vi "GeoData.vi"() -> ()   [LabVIEW 2017] (continued)
31003\tClearwater\tNE\tAntelope County\tH1\n68764\t31003\tOrchard\tNE\tAntelope County\tH1\n68636\t31003\tElgin\tNE\tAntelope County\tH1\n68735\t31003\tEwing\tNE\tAntelope County\tH1\n68773\t31003\tRoyal\tNE\tAntelope County\tH1\n68761\t31003\tOakdale\tNE\tAntelope County\tH1\n68756\t31003\tNeligh\tNE\tAntelope County\tH1\n68729\t31003\tCreighton\tNE\tAntelope County\tH1\n69121\t31005\tArthur\tNE\tArthur County\tH1\n69146\t31005\tLemoyne\tNE\tArthur County\tH1\n69350\t31005\tHyannis\tNE\tArthur County\tH1\n69165\t31005\tSutherland\tNE\tArthur County\tH1\n69147\t31005\tLewellen\tNE\tArthur County\tH1\n69144\t31005\tKeystone\tNE\tArthur County\tH1\n69366\t31005\tWhitman\tNE\tArthur County\tH1\n69156\t31007\tPotter\tNE\tBanner County\tH1\n69145\t31007\tKimball\tNE\tBanner County\tH1\n69345\t31007\tHarrisburg\tNE\tBanner County\tH1\n69334\t31007\tBayard\tNE\tBanner County\tH1\n68833\t31009\tDunning\tNE\tBlaine County\tH1\n69157\t31009\tPurdum\tNE\tBlaine County\tH1\n68821\t31009\tBrewster\tNE\tBlaine County\tH1\n69163\t31009\tStapleton\tNE\tBlaine County\tH1\n69142\t31009\tHalsey\tNE\tBlaine County\tH1\n68781\t31011\tTilden\tNE\tBoone County\tH1\n68652\t31011\tPetersburg\tNE\tBoone County\tH1\n68655\t31011\tPrimrose\tNE\tBoone County\tH1\n68623\t31011\tBelgrade\tNE\tBoone County\tH1\n68660\t31011\tSaint edward\tNE\tBoone County\tH1\n68620\t31011\tAlbion\tNE\tBoone County\tH1\n68636\t31011\tElgin\tNE\tBoone County\tH1\n68638\t31011\tFullerton\tNE\tBoone County\tH1\n68627\t31011\tCedar rapids\tNE\tBoone County\tH1\n68758\t31011\tNewman grove\tNE\tBoone County\tH1\n68882\t31011\tWolbach\tNE\tBoone County\tH1\n69301\t31013\tAlliance\tNE\tBox Butte County\tH1\n69348\t31013\tHemingford\tNE\tBox Butte County\tH1\n69354\t31013\tMarsland\tNE\tBox Butte County\tH1\n68746\t31015\tLynch\tNE\tBoyd County\tH1\n68755\t31015\tNaper\tNE\tBoyd County\tH1\n68777\t31015\tSpencer\tNE\tBoyd County\tH1\n68722\t31015\tButte\tNE\tBoyd County\tH1\n68719\t31015\tBristow\tNE\tBoyd County\tH1\n68714\t31017\tBassett\tNE\tBrown County\tH1\n69210\t31017\tAinsworth\tNE\tBrown County\tH1\n69217\t31017\tLong pine\tNE\tBrown County\tH1\n69135\t31017\tElsmere\tNE\tBrown County\tH1\n69214\t31017\tJohnstown\tNE\tBrown County\tH1\n69221\t31017\tWood lake\tNE\tBrown County\tH1\n68847\t31019\tKearney\tNE\tBuffalo County\tH1\n68844\t31019\tHazard\tNE\tBuffalo County\tH1\n68956\t31019\tKenesaw\tNE\tBuffalo County\tH1\n68866\t31019\tPleasanton\tNE\tBuffalo County\tH1\n68947\t31019\tHildreth\tNE\tBuffalo County\tH1\n68845\t31019\tKearney\tNE\tBuffalo County\tH1\n68836\t31019\tElm creek\tNE\tBuffalo County\tH1\n68855\t31019\tMason city\tNE\tBuffalo County\tH1\n68876\t31019\tShelton\tNE\tBuffalo County\tH1\n68861\t31019\tOdessa\tNE\tBuffalo County\tH1\n68870\t31019\tRiverdale\tNE\tBuffalo County\tH1\n68840\t31019\tGibbon\tNE\tBuffalo County\tH1\n68849\t31019\tKearney\tNE\tBuffalo County\tH1\n68869\t31019\tRavenna\tNE\tBuffalo County\tH1\n68848\t31019\tKearney\tNE\tBuffalo County\tH1\n68858\t31019\tMiller\tNE\tBuffalo County\tH1\n68812\t31019\tAmherst\tNE\tBuffalo County\tH1\n68029\t31021\tHerman\tNE\tBurt County\tH1\n68019\t31021\tCraig\tNE\tBurt County\tH1\n68004\t31021\tBancroft\tNE\tBurt County\tH1\n68061\t31021\tTekamah\tNE\tBurt County\tH1\n68045\t31021\tOakland\tNE\tBurt County\tH1\n68031\t31021\tHooper\tNE\tBurt County\tH1\n68038\t31021\tLyons\tNE\tBurt County\tH1\n68020\t31021\tDecatur\tNE\tBurt County\tH1\n68036\t31023\tLinwood\tNE\tButler County\tH1\n68601\t31023\tColumbus\tNE\tButler County\tH1\n68626\t31023\tBrainard\tNE\tButler County\tH1\n68014\t31023\tBruno\tNE\tButler County\tH1\n68635\t31023\tDwight\tNE\tButler County\tH1\n68632\t31023\tDavid city\tNE\tButler County\tH1\n68658\t31023\tRising city\tNE\tButler County\tH1\n68669\t31023\tUlysses\tNE\tButler County\tH1\n68314\t31023\tBee\tNE\tButler County\tH1\n68662\t31023\tShelby\tNE\tButler County\tH1\n68001\t31023\tAbie\tNE\tButler County\tH1\n68624\t31023\tBellwood\tNE\tButler County\tH1\n68667\t31023\tSurprise\tNE\tButler County\tH1\n68349\t31025\tElmwood\tNE\tCass County\tH1\n68407\t31025\tMurdock\tNE\tCass County\tH1\n68016\t31025\tCedar creek\tNE\tCass County\tH1\n68037\t31025\tLouisville\tNE\tCass County\tH1\n68403\t31025\tManley\tNE\tCass County\tH1\n68347\t31025\tEagle\tNE\tCass County\tH1\n68454\t31025\tUnadilla\tNE\tCass County\tH1\n68058\t31025\tSouth bend\tNE\tCass County\tH1\n68048\t31025\tPlattsmouth\tNE\tCass County\tH1\n68527\t31025\tLincoln\tNE\tCass County\tH1\n68003\t31025\tAshland\tNE\tCass County\tH1\n68462\t31025\tWaverly\tNE\tCass County\tH1\n68304\t31025\tAlvo\tNE\tCass County\tH1\n68413\t31025\tNehawka\tNE\tCass County\tH1\n68455\t31025\tUnion\tNE\tCass County\tH1\n68418\t31025\tPalmyra\tNE\tCass County\tH1\n68307\t31025\tAvoca\tNE\tCass County\tH1\n68463\t31025\tWeeping water\tNE\tCass County\tH1\n68366\t31025\tGreenwood\tNE\tCass County\tH1\n68409\t31025\tMurray\tNE\tCass County\tH1\n68745\t31027\tLaurel\tNE\tCedar County\tH1\n68736\t31027\tFordyce\tNE\tCedar County\tH1\n68717\t31027\tBelden\tNE\tCedar County\tH1\n68786\t31027\tWausa\tNE\tCedar County\tH1\n68727\t31027\tColeridge\tNE\tCedar County\tH1\n68757\t31027\tNewcastle\tNE\tCedar County\tH1\n68739\t31027\tHartington\tNE\tCedar County\tH1\n68749\t31027\tMagnet\tNE\tCedar County\tH1\n68792\t31027\tWynot\tNE\tCedar County\tH1\n68771\t31027\tRandolph\tNE\tCedar County\tH1\n68774\t31027\tSaint helena\tNE\tCedar County\tH1\n68718\t31027\tBloomfield\tNE\tCedar County\tH1\n68730\t31027\tCrofton\tNE\tCedar County\tH1\n69027\t31029\tEnders\tNE\tChase County\tH1\n69030\t31029\tHaigler\tNE\tChase County\tH1\n69134\t31029\tElsie\tNE\tChase County\tH1\n69045\t31029\tWauneta\tNE\tChase County\tH1\n69033\t31029\tImperial\tNE\tChase County\tH1\n69023\t31029\tChampion\tNE\tChase County\tH1\n69168\t31029\tVenango\tNE\tChase County\tH1\n69343\t31031\tGordon\tNE\tCherry County\tH1\n69166\t31031\tThedford\tNE\tCherry County\tH1\n69212\t31031\tCrookston\tNE\tCherry County\tH1\n69211\t31031\tCody\tNE\tCherry County\tH1\n69350\t31031\tHyannis\tNE\tCherry County\tH1\n69219\t31031\tNenzel\tNE\tCherry County\tH1\n69220\t31031\tSparks\tNE\tCherry County\tH1\n69333\t31031\tAshby\tNE\tCherry County\tH1\n69161\t31031\tSeneca\tNE\tCherry County\tH1\n69201\t31031\tValentine\tNE\tCherry County\tH1\n69216\t31031\tKilgore\tNE\tCherry County\tH1\n69218\t31031\tMerriman\tNE\tCherry County\tH1\n69366\t31031\tWhitman\tNE\tCherry County\tH1\n69221\t31031\tWood lake\tNE\tCherry County\tH1\n69156\t31033\tPotter\tNE\tCheyenne County\tH1\n69149\t31033\tLodgepole\tNE\tCheyenne County\tH1\n69162\t31033\tSidney\tNE\tCheyenne County\tH1\n69141\t31033\tGurley\tNE\tCheyenne County\tH1\n69131\t31033\tDalton\tNE\tCheyenne County\tH1\n68436\t31035\tShickley\tNE\tClay County\tH1\n68452\t31035\tOng\tNE\tClay County\tH1\n68944\t31035\tHarvard\tNE\tClay County\tH1\n68933\t31035\tClay center\tNE\tClay County\tH1\n68935\t31035\tEdgar\tNE\tClay County\tH1\n68930\t31035\tBlue hill\tNE\tClay County\tH1\n68818\t31035\tAurora\tNE\tClay County\tH1\n68979\t31035\tSutton\tNE\tClay County\tH1\n68934\t31035\tDeweese\tNE\tClay County\tH1\n68901\t31035\tHastings\tNE\tClay County\tH1\n68941\t31035\tGlenvil\tNE\tClay County\tH1\n68975\t31035\tSaronville\tNE\tClay County\tH1\n68938\t31035\tFairfield\tNE\tClay County\tH1\n68954\t31035\tInland\tNE\tClay County\tH1\n68980\t31035\tTrumbull\tNE\tClay County\tH1\n68601\t31037\tColumbus\tNE\tColfax County\tH1\n68641\t31037\tHowells\tNE\tColfax County\tH1\n68659\t31037\tRogers\tNE\tColfax County\tH1\n68661\t31037\tSchuyler\tNE\tColfax County\tH1\n68643\t31037\tLeigh\tNE\tColfax County\tH1\n68633\t31037\tDodge\tNE\tColfax County\tH1\n68629\t31037\tClarkson\tNE\tColfax County\tH1\n68047\t31039\tPender\tNE\tCuming County\tH1\n68641\t31039\tHowells\tNE\tCuming County\tH1\n68004\t31039\tBancroft\tNE\tCuming County\tH1\n68045\t31039\tOakland\tNE\tCuming County\tH1\n68788\t31039\tWest point\tNE\tCuming County\tH1\n68716\t31039\tBeemer\tNE\tCuming County\tH1\n68768\t31039\tPilger\tNE\tCuming County\tH1\n68791\t31039\tWisner\tNE\tCuming County\tH1\n68633\t31039\tDodge\tNE\tCuming County\tH1\n68038\t31039\tLyons\tNE\tCuming County\tH1\n68825\t31041\tCallaway\tNE\tCuster County\tH1\n68856\t31041\tMerna\tNE\tCuster County\tH1\n69138\t31041\tGothenburg\tNE\tCuster County\tH1\n68833\t31041\tDunning\tNE\tCuster County\tH1\n68866\t31041\tPleasanton\tNE\tCuster County\tH1\n68815\t31041\tArcadia\tNE\tCuster County\tH1\n68860\t31041\tOconto\tNE\tCuster County\tH1\n68855\t31041\tMason city\tNE\tCuster County\tH1\n68881\t31041\tWesterville\tNE\tCuster County\tH1\n68874\t31041\tSargent\tNE\tCuster County\tH1\n68834\t31041\tEddyville\tNE\tCuster County\tH1\n68813\t31041\tAnselmo\tNE\tCuster County\tH1\n68850\t31041\tLexington\tNE\tCuster County\tH1\n68814\t31041\tAnsley\tNE\tCuster County\tH1\n68878\t31041\tSumner\tNE\tCuster County\tH1\n69120\t31041\tArnold\tNE\tCuster County\tH1\n68823\t31041\tBurwell\tNE\tCuster County\tH1\n68852\t31041\tLitchfield\tNE\tCuster County\tH1\n68822\t31041\tBroken bow\tNE\tCuster County\tH1\n68828\t31041\tComstock\tNE\tCuster County\tH1\n68030\t31043\tHomer\tNE\tDakota County\tH1\n68741\t31043\tHubbard\tNE\tDakota County\tH1\n68731\t31043\tDakota city\tNE\tDakota County\tH1\n68770\t31043\tPonca\tNE\tDakota County\tH1\n68733\t31043\tEmerson\tNE\tDakota County\tH1\n68776\t31043\tSouth sioux city\tNE\tDakota County\tH1\n68743\t31043\tJackson\tNE\tDakota County\tH1\n68785\t31043\tWaterbury\tNE\tDakota County\tH1\n69348\t31045\tHemingford\tNE\tDawes County\tH1\n69337\t31045\tChadron\tNE\tDawes County\tH1\n69347\t31045\tHay springs\tNE\tDawes County\tH1\n69339\t31045\tCrawford\tNE\tDawes County\tH1\n69367\t31045\tWhitney\tNE\tDawes County\tH1\n69354\t31045\tMarsland\tNE\tDawes County\tH1\n69029\t31047\tFarnam\tNE\tDawson County\tH1\n69138\t31047\tGothenburg\tNE\tDawson County\tH1\n68836\t31047\tElm creek\tNE\tDawson County\tH1\n69130\t31047\tCozad\tNE\tDawson County\tH1\n69171\t31047\tWillow island\tNE\tDawson County\tH1\n68834\t31047\tEddyville\tNE\tDawson County\tH1\n69028\t31047\tEustis\tNE\tDawson County\tH1\n68850\t31047\tLexington\tNE\tDawson County\tH1\n68878\t31047\tSumner\tNE\tDawson County\tH1\n68863\t31047\tOverton\tNE\tDawson County\tH1\n68937\t31047\tElwood\tNE\tDawson County\tH1\n68858\t31047\tMiller\tNE\tDawson County\tH1\n69129\t31049\tChappell\tNE\tDeuel County\tH1\n69149\t31049\tLodgepole\tNE\tDeuel County\tH1\n69122\t31049\tBig springs\tNE\tDeuel County\tH1\n68745\t31051\tLaurel\tNE\tDixon County\tH1\n68757\t31051\tNewcastle\tNE\tDixon County\tH1\n68739\t31051\tHartington\tNE\tDixon County\tH1\n68770\t31051\tPonca\tNE\tDixon County\tH1\n68733\t31051\tEmerson\tNE\tDixon County\tH1\n68732\t31051\tDixon\tNE\tDixon County\tH1\n68792\t31051\tWynot\tNE\tDixon County\tH1\n68787\t31051\tWayne\tNE\tDixon County\tH1\n68710\t31051\tAllen\tNE\tDixon County\tH1\n68728\t31051\tConcord\tNE\tDixon County\tH1\n68784\t31051\tWakefield\tNE\tDixon County\tH1\n68785\t31051\tWaterbury\tNE\tDixon County\tH1\n68751\t31051\tMaskell\tNE\tDixon County\tH1\n68063\t31053\tUehling\tNE\tDodge County\tH1\n68026\t31053\tFremont\tNE\tDodge County\tH1\n68044\t31053\tNickerson\tNE\tDodge County\tH1\n68064\t31053\tValley\tNE\tDodge County\tH1\n68045\t31053\tOakland\tNE\tDodge County\tH1\n68649\t31053\tNorth bend\tNE\tDodge County\tH1\n68788\t31053\tWest point\tNE\tDodge County\tH1\n68664\t31053\tSnyder\tNE\tDodge County\tH1\n68025\t31053\tFremont\tNE\tDodge County\tH1\n68621\t31053\tAmes\tNE\tDodge County\tH1\n68031\t31053\tHooper\tNE\tDodge County\tH1\n68072\t31053\tWinslow\tNE\tDodge County\tH1\n68633\t31053\tDodge\tNE\tDodge County\tH1\n68057\t31053\tScribner\tNE\tDodge County\tH1\n68118\t31055\tOmaha\tNE\tDouglas County\tH1\n68106\t31055\tOmaha\tNE\tDouglas County\tH1\n68022\t31055\tElkhorn\tNE\tDouglas County\tH1\n68135\t31055\tOmaha\tNE\tDouglas County\tH1\n68117\t31055\tOmaha\tNE\tDouglas County\tH1\n68108\t31055\tOmaha\tNE\tDouglas County\tH1\n68137\t31055\tOmaha\tNE\tDouglas County\tH1\n68154\t31055\tOmaha\tNE\tDouglas County\tH1\n68152\t31055\tOmaha\tNE\tDouglas County\tH1\n68007\t31055\tBennington\tNE\tDouglas County\tH1\n68182\t31055\tOmaha\tNE\tDouglas County\tH1\n68112\t31055\tOmaha\tNE\tDouglas County\tH1\n68114\t31055\tOmaha\tNE\tDouglas County\tH1\n68116\t31055\tOmaha\tNE\tDouglas County\tH1\n68127\t31055\tOmaha\tNE\tDouglas County\tH1\n68138\t31055\tOmaha\tNE\tDouglas County\tH1\n68197\t31055\tOmaha\tNE\tDouglas County\tH1\n68145\t31055\tOmaha\tNE\tDouglas County\tH1\n68179\t31055\tOmaha\tNE\tDouglas County\tH1\n68139\t31055\tOmaha\tNE\tDouglas County\tH1\n68175\t31055\tOmaha\tNE\tDouglas County\tH1\n68122\t31055\tOmaha\tNE\tDouglas County\tH1\n68102\t31055\tOmaha\tNE\tDouglas County\tH1\n68064\t31055\tValley\tNE\tDouglas County\tH1\n68136\t31055\tOmaha\tNE\tDouglas County\tH1\n68069\t31055\tWaterloo\tNE\tDouglas County\tH1\n68198\t31055\tOmaha\tNE\tDouglas County\tH1\n68111\t31055\tOmaha\tNE\tDouglas County\tH1\n68144\t31055\tOmaha\tNE\tDouglas County\tH1\n68130\t31055\tOmaha\tNE\tDouglas County\tH1\n68109\t31055\tOmaha\tNE\tDouglas County\tH1\n68134\t31055\tOmaha\tNE\tDouglas County\tH1\n68107\t31055\tOmaha\tNE\tDouglas County\tH1\n68110\t31055\tOmaha\tNE\tDouglas County\tH1\n68131\t31055\tOmaha\tNE\tDouglas County\tH1\n68147\t31055\tBellevue\tNE\tDouglas County\tH1\n68010\t31055\tBoys town\tNE\tDouglas County\tH1\n68180\t31055\tOmaha\tNE\tDouglas County\tH1\n68178\t31055\tOmaha\tNE\tDouglas County\tH1\n68105\t31055\tOmaha\tNE\tDouglas County\tH1\n68124\t31055\tOmaha\tNE\tDouglas County\tH1\n68132\t31055\tOmaha\tNE\tDouglas County\tH1\n68142\t31055\tOmaha\tNE\tDouglas County\tH1\n68103\t31055\tOmaha\tNE\tDouglas County\tH1\n68028\t31055\tGretna\tNE\tDouglas County\tH1\n68104\t31055\tOmaha\tNE\tDouglas County\tH1\n68128\t31055\tLa vista\tNE\tDouglas County\tH1\n68164\t31055\tOmaha\tNE\tDouglas County\tH1\n68157\t31055\tOmaha\tNE\tDouglas County\tH1\n68183\t31055\tOmaha\tNE\tDouglas County\tH1\n69037\t31057\tMax\tNE\tDundy County\tH1\n69027\t31057\tEnders\tNE\tDundy County\tH1\n69030\t31057\tHaigler\tNE\tDundy County\tH1\n69045\t31057\tWauneta\tNE\tDundy County\tH1\n69021\t31057\tBenkelman\tNE\tDundy County\tH1\n69041\t31057\tParks\tNE\tDundy County\tH1\n68436\t31059\tShickley\tNE\tFillmore County\tH1\n68452\t31059\tOng\tNE\tFillmore County\tH1\n68444\t31059\tStrang\tNE\tFillmore County\tH1\n68416\t31059\tOhiowa\tNE\tFillmore County\tH1\n68326\t31059\tCarleton\tNE\tFillmore County\tH1\n68406\t31059\tMilligan\tNE\tFillmore County\tH1\n68361\t31059\tGeneva\tNE\tFillmore County\tH1\n68359\t31059\tFriend\tNE\tFillmore County\tH1\n68351\t31059\tExeter\tNE\tFillmore County\tH1\n68354\t31059\tFairmont\tNE\tFillmore County\tH1\n68979\t31059\tSutton\tNE\tFillmore County\tH1\n68365\t31059\tGrafton\tNE\tFillmore County\tH1\n68322\t31059\tBruning\tNE\tFillmore County\tH1\n68335\t31059\tDavenport\tNE\tFillmore County\tH1\n68972\t31061\tRiverton\tNE\tFranklin County\tH1\n68947\t31061\tHildreth\tNE\tFranklin County\tH1\n68939\t31061\tFranklin\tNE\tFranklin County\tH1\n68981\t31061\tUpland\tNE\tFranklin County\tH1\n68982\t31061\tWilcox\tNE\tFranklin County\tH1\n68960\t31061\tNaponee\tNE\tFranklin County\tH1\n68932\t31061\tCampbell\tNE\tFranklin County\tH1\n68952\t31061\tInavale\tNE\tFranklin County\tH1\n68929\t31061\tBloomington\tNE\tFranklin County\tH1\n69029\t31063\tFarnam\tNE\tFrontier County\tH1\n69038\t31063\tMaywood\tNE\tFrontier County\tH1\n69039\t31063\tMoorefield\tNE\tFrontier County\tH1\n69001\t31063\tMc cook\tNE\tFrontier County\tH1\n69022\t31063\tCambridge\tNE\tFrontier County\tH1\n69028\t31063\tEustis\tNE\tFrontier County\tH1\n68948\t31063\tHolbrook\tNE\tFrontier County\tH1\n69025\t31063\tCurtis\tNE\tFrontier County\tH1\n69042\t31063\tStockville\tNE\tFrontier County\tH1\n69034\t31063\tIndianola\tNE\tFrontier County\tH1\n68922\t31065\tArapahoe\tNE\tFurnas County\tH1\n68977\t31065\tStamford\tNE\tFurnas County\tH1\n68936\t31065\tEdison\tNE\tFurnas County\tH1\n69022\t31065\tCambridge\tNE\tFurnas County\tH1\n69046\t31065\tWilsonville\tNE\tFurnas County\tH1\n68967\t31065\tOxford\tNE\tFurnas County\tH1\n69020\t31065\tBartley\tNE\tFurnas County\tH1\n68926\t31065\tBeaver city\tNE\tFurnas County\tH1\n68948\t31065\tHolbrook\tNE\tFurnas County\tH1\n68946\t31065\tHendley\tNE\tFurnas County\tH1\n68309\t31067\tBarneston\tNE\tGage County\tH1\n68301\t31067\tAdams\tNE\tGage County\tH1\n68458\t31067\tVirginia\tNE\tGage County\tH1\n68331\t31067\tCortland\tNE\tGage County\tH1\n68342\t31067\tDiller\tNE\tGage County\tH1\n68422\t31067\tPickrell\tNE\tGage County\tH1\n68323\t31067\tBurchard\tNE\tGage County\tH1\n68466\t31067\tWymore\tNE\tGage County\tH1\n68368\t31067\tHallam\tNE\tGage County\tH1\n68381\t31067\tLiberty\tNE\tGage County\tH1\n68328\t31067\tClatonia\tNE\tGage County\tH1\n68341\t31067\tDe witt\tNE\tGage County\tH1\n68404\t31067\tMartell\tNE\tGage County\tH1\n68332\t31067\tCrab orchard\tNE\tGage County\tH1\n68415\t31067\tOdell\tNE\tGage County\tH1\n68465\t31067\tWilber\tNE\tGage County\tH1\n68358\t31067\tFirth\tNE\tGage County\tH1\n68310\t31067\tBeatrice\tNE\tGage County\tH1\n68318\t31067\tBlue springs\tNE\tGage County\tH1\n68424\t31067\tPlymouth\tNE\tGage County\tH1\n68357\t31067\tFilley\tNE\tGage County\tH1\n69129\t31069\tChappell\tNE\tGarden County\tH1\n69351\t31069\tLakeside\tNE\tGarden County\tH1\n69335\t31069\tBingham\tNE\tGarden County\tH1\n69149\t31069\tLodgepole\tNE\tGarden County\tH1\n69333\t31069\tAshby\tNE\tGarden County\tH1\n69148\t31069\tLisco\tNE\tGarden County\tH1\n69190\t31069\tOshkosh\tNE\tGarden County\tH1\n69147\t31069\tLewellen\tNE\tGarden County\tH1\n69154\t31069\tOshkosh\tNE\tGarden County\tH1\n69122\t31069\tBig springs\tNE\tGarden County\tH1\n69340\t31069\tEllsworth\tNE\tGarden County\tH1\n68725\t31071\tChambers\tNE\tGarfield County\tH1\n68862\t31071\tOrd\tNE\tGarfield County\tH1\n68823\t31071\tBurwell\tNE\tGarfield County\tH1\n68637\t31071\tEricson\tNE\tGarfield County\tH1\n68922\t31073\tArapahoe\tNE\tGosper County\tH1\n68936\t31073\tEdison\tNE\tGosper County\tH1\n69022\t31073\tCambridge\tNE\tGosper County\tH1\n68967\t31073\tOxford\tNE\tGosper County\tH1\n69028\t31073\tEustis\tNE\tGosper County\tH1\n68850\t31073\tLexington\tNE\tGosper County\tH1\n68937\t31073\tElwood\tNE\tGosper County\tH1\n68948\t31073\tHolbrook\tNE\tGosper County\tH1\n68927\t31073\tBertrand\tNE\tGosper County\tH1\n68976\t31073\tSmithfield\tNE\tGosper County\tH1\n69350\t31075\tHyannis\tNE\tGrant County\tH1\n69333\t31075\tAshby\tNE\tGrant County\tH1\n69366\t31075\tWhitman\tNE\tGrant County\tH1\n68835\t31077\tElba\tNE\tGreeley County\tH1\n68665\t31077\tSpalding\tNE\tGreeley County\tH1\n68655\t31077\tPrimrose\tNE\tGreeley County\tH1\n68842\t31077\tGreeley\tNE\tGreeley County\tH1\n68875\t31077\tScotia\tNE\tGreeley County\tH1\n68637\t31077\tEricson\tNE\tGreeley County\tH1\n68859\t31077\tNorth loup\tNE\tGreeley County\tH1\n68627\t31077\tCedar rapids\tNE\tGreeley County\tH1\n68882\t31077\tWolbach\tNE\tGreeley County\tH1\n68955\t31079\tJuniata\tNE\tHall County\tH1\n68956\t31079\tKenesaw\tNE\tHall County\tH1\n68831\t31079\tDannebrog\tNE\tHall County\tH1\n68876\t31079\tShelton\tNE\tHall County\tH1\n68865\t31079\tPhillips\tNE\tHall County\tH1\n68832\t31079\tDoniphan\tNE\tHall County\tH1\n68810\t31079\tAlda\tNE\tHall County\tH1\n68883\t31079\tWood river\tNE\tHall County\tH1\n68803\t31079\tGrand island\tNE\tHall County\tH1\n68802\t31079\tGrand island\tNE\tHall County\tH1\n68901\t31079\tHastings\tNE\tHall County\tH1\n68824\t31079\tCairo\tNE\tHall County\tH1\n68869\t31079\tRavenna\tNE\tHall County\tH1\n68872\t31079\tSaint libory\tNE\tHall County\tH1\n68801\t31079\tGrand island\tNE\tHall County\tH1\n68980\t31079\tTrumbull\tNE\tHall County\tH1\n68654\t31081\tPolk\tNE\tHamilton County\tH1\n68944\t31081\tHarvard\tNE\tHamilton County\tH1\n68854\t31081\tMarquette\tNE\tHamilton County\tH1\n68628\t31081\tClarks\tNE\tHamilton County\tH1\n68371\t31081\tHenderson\tNE\tHamilton County\tH1\n68865\t31081\tPhillips\tNE\tHamilton County\tH1\n68832\t31081\tDoniphan\tNE\tHamilton County\tH1\n68846\t31081\tHordville\tNE\tHamilton County\tH1\n68841\t31081\tGiltner\tNE\tHamilton County\tH1\n68319\t31081\tBradshaw\tNE\tHamilton County\tH1\n68818\t31081\tAurora\tNE\tHamilton County\tH1\n68979\t31081\tSutton\tNE\tHamilton County\tH1\n68843\t31081\tHampton\tNE\tHamilton County\tH1\n68980\t31081\tTrumbull\tNE\tHamilton County\tH1\n68977\t31083\tStamford\tNE\tHarlan County\tH1\n68949\t31083\tHoldrege\tNE\tHarlan County\tH1\n68967\t31083\tOxford\tNE\tHarlan County\tH1\n68920\t31083\tAlma\tNE\tHarlan County\tH1\n68982\t31083\tWilcox\tNE\tHarlan County\tH1\n68960\t31083\tNaponee\tNE\tHarlan County\tH1\n68966\t31083\tOrleans\tNE\tHarlan County\tH1\n68971\t31083\tRepublican city\tNE\tHarlan County\tH1\n68969\t31083\tRagan\tNE\tHarlan County\tH1\n69038\t31085\tMaywood\tNE\tHayes County\tH1\n69024\t31085\tCulbertson\tNE\tHayes County\tH1\n69169\t31085\tWallace\tNE\tHayes County\tH1\n69032\t31085\tHayes center\tNE\tHayes County\tH1\n69134\t31085\tElsie\tNE\tHayes County\tH1\n69045\t31085\tWauneta\tNE\tHayes County\tH1\n69040\t31085\tPalisade\tNE\tHayes County\tH1\n69038\t31087\tMaywood\tNE\tHitchcock County\tH1\n69024\t31087\tCulbertson\tNE\tHitchcock County\tH1\n69043\t31087\tStratton\tNE\tHitchcock County\tH1\n69001\t31087\tMc cook\tNE\tHitchcock County\tH1\n69045\t31087\tWauneta\tNE\tHitchcock County\tH1\n69040\t31087\tPalisade\tNE\tHitchcock County\tH1\n69044\t31087\tTrenton\tNE\tHitchcock County\tH1\n68766\t31089\tPage\tNE\tHolt County\tH1\n68759\t31089\tNewport\tNE\tHolt County\tH1\n68725\t31089\tChambers\tNE\tHolt County\tH1\n68713\t31089\tAtkinson\tNE\tHolt County\tH1\n68746\t31089\tLynch\tNE\tHolt County\tH1\n68726\t31089\tClearwater\tNE\tHolt County\tH1\n68823\t31089\tBurwell\tNE\tHolt County\tH1\n68764\t31089\tOrchard\tNE\tHolt County\tH1\n68735\t31089\tEwing\tNE\tHolt County\tH1\n68763\t31089\tOneill\tNE\tHolt County\tH1\n68711\t31089\tAmelia\tNE\tHolt County\tH1\n68777\t31089\tSpencer\tNE\tHolt County\tH1\n68780\t31089\tStuart\tNE\tHolt County\tH1\n68734\t31089\tEmmet\tNE\tHolt County\tH1\n68742\t31089\tInman\tNE\tHolt County\tH1\n69152\t31091\tMullen\tNE\tHooker County\tH1\n69167\t31091\tTryon\tNE\tHooker County\tH1\n68873\t31093\tSaint paul\tNE\tHoward County\tH1\n68816\t31093\tArcher\tNE\tHoward County\tH1\n68835\t31093\tElba\tNE\tHoward County\tH1\n68831\t31093\tDannebrog\tNE\tHoward County\tH1\n68817\t31093\tAshton\tNE\tHoward County\tH1\n68864\t31093\tPalmer\tNE\tHoward County\tH1\n68875\t31093\tScotia\tNE\tHoward County\tH1\n68838\t31093\tFarwell\tNE\tHoward County\tH1\n68803\t31093\tGrand island\tNE\tHoward County\tH1\n68824\t31093\tCairo\tNE\tHoward County\tH1\n68872\t31093\tSaint libory\tNE\tHoward County\tH1\n68801\t31093\tGrand island\tNE\tHoward County\tH1\n68882\t31093\tWolbach\tNE\tHoward County\tH1\n68820\t31093\tBoelus\tNE\tHoward County\tH1\n68352\t31095\tFairbury\tNE\tJefferson County\tH1\n68464\t31095\tWestern\tNE\tJefferson County\tH1\n68350\t31095\tEndicott\tNE\tJefferson County\tH1\n68342\t31095\tDiller\tNE\tJefferson County\tH1\n68440\t31095\tSteele city\tNE\tJefferson County\tH1\n68303\t31095\tAlexandria\tNE\tJefferson County\tH1\n68429\t31095\tReynolds\tNE\tJefferson County\tH1\n68341\t31095\tDe witt\tNE\tJefferson County\tH1\n68370\t31095\tHebron\tNE\tJefferson County\tH1\n68453\t31095\tTobias\tNE\tJefferson County\tH1\n68310\t31095\tBeatrice\tNE\tJefferson County\tH1\n68424\t31095\tPlymouth\tNE\tJefferson County\tH1\n68338\t31095\tDaykin\tNE\tJefferson County\tH1\n68377\t31095\tJansen\tNE\tJefferson County\tH1\n68301\t31097\tAdams\tNE\tJohnson County\tH1\n68378\t31097\tJohnson\tNE\tJohnson County\tH1\n68329\t31097\tCook\tNE\tJohnson County\tH1\n68443\t31097\tSterling\tNE\tJohnson County\tH1\n68450\t31097\tTecumseh\tNE\tJohnson County\tH1\n68324\t31097\tBurr\tNE\tJohnson County\tH1\n68332\t31097\tCrab orchard\tNE\tJohnson County\tH1\n68447\t31097\tTable rock\tNE\tJohnson County\tH1\n68348\t31097\tElk creek\tNE\tJohnson County\tH1\n68448\t31097\tTalmage\tNE\tJohnson County\tH1\n68847\t31099\tKearney\tNE\tKearney County\tH1\n68956\t31099\tKenesaw\tNE\tKearney County\tH1\n68972\t31099\tRiverton\tNE\tKearney County\tH1\n68945\t31099\tHeartwell\tNE\tKearney County\tH1\n68947\t31099\tHildreth\tNE\tKearney County\tH1\n68845\t31099\tKearney\tNE\tKearney County\tH1\n68924\t31099\tAxtell\tNE\tKearney County\tH1\n68939\t31099\tFranklin\tNE\tKearney County\tH1\n68981\t31099\tUpland\tNE\tKearney County\tH1\n68840\t31099\tGibbon\tNE\tKearney County\tH1\n68982\t31099\tWilcox\tNE\tKearney County\tH1\n68959\t31099\tMinden\tNE\tKearney County\tH1\n68932\t31099\tCampbell\tNE\tKearney County\tH1\n69121\t31101\tArthur\tNE\tKeith County\tH1\n69155\t31101\tPaxton\tNE\tKeith County\tH1\n69146\t31101\tLemoyne\tNE\tKeith County\tH1\n69153\t31101\tOgallala\tNE\tKeith County\tH1\n69165\t31101\tSutherland\tNE\tKeith County\tH1\n69147\t31101\tLewellen\tNE\tKeith County\tH1\n69144\t31101\tKeystone\tNE\tKeith County\tH1\n69127\t31101\tBrule\tNE\tKeith County\tH1\n69122\t31101\tBig springs\tNE\tKeith County\tH1\n68753\t31103\tMills\tNE\tKeya Paha County\tH1\n68778\t31103\tSpringview\tNE\tKeya Paha County\tH1\n69156\t31105\tPotter\tNE\tKimball County\tH1\n69145\t31105\tKimball\tNE\tKimball County\tH1\n69133\t31105\tDix\tNE\tKimball County\tH1\n69128\t31105\tBushnell\tNE\tKimball County\tH1\n68760\t31107\tNiobrara\tNE\tKnox County\tH1\n68769\t31107\tPlainview\tNE\tKnox County\tH1\n68786\t31107\tWausa\tNE\tKnox County\tH1\n68724\t31107\tCenter\tNE\tKnox County\tH1\n68789\t31107\tWinnetoon\tNE\tKnox County\tH1\n68783\t31107\tVerdigre\tNE\tKnox County\tH1\n68764\t31107\tOrchard\tNE\tKnox County\tH1\n68773\t31107\tRoyal\tNE\tKnox County\tH1\n68763\t31107\tOneill\tNE\tKnox County\tH1\n68718\t31107\tBloomfield\tNE\tKnox County\tH1\n68730\t31107\tCrofton\tNE\tKnox County\tH1\n68729\t31107\tCreighton\tNE\tKnox County\tH1\n68503\t31109\tLincoln\tNE\tLancaster County\tH1\n68428\t31109\tRaymond\tNE\tLancaster County\tH1\n68526\t31109\tLincoln\tNE\tLancaster County\tH1\n68301\t31109\tAdams\tNE\tLancaster County\tH1\n68419\t31109\tPanama\tNE\tLancaster County\tH1\n68017\t31109\tCeresco\tNE\tLancaster County\tH1\n68331\t31109\tCortland\tNE\tLancaster County\tH1\n68522\t31109\tLincoln\tNE\tLancaster County\tH1\n68523\t31109\tLincoln\tNE\tLancaster County\tH1\n68438\t31109\tSprague\tNE\tLancaster County\tH1\n68501\t31109\tLincoln\tNE\tLancaster County\tH1\n68339\t31109\tDenton\tNE\tLancaster County\tH1\n68360\t31109\tGarland\tNE\tLancaster County\tH1\n68065\t31109\tValparaiso\tNE\tLancaster County\tH1\n68502\t31109\tLincoln\tNE\tLancaster County\tH1\n68507\t31109\tLincoln\tNE\tLancaster County\tH1\n68423\t31109\tPleasant dale\tNE\tLancaster County\tH1\n68516\t31109\tLincoln\tNE\tLancaster County\tH1\n68528\t31109\tLincoln\tNE\tLancaster County\tH1\n68588\t31109\tLincoln\tNE\tLancaster County\tH1\n68347\t31109\tEagle\tNE\tLancaster County\tH1\n68368\t31109\tHallam\tNE\tLancaster County\tH1\n68506\t31109\tLincoln\tNE\tLancaster County\tH1\n68510\t31109\tLincoln\tNE\tLancaster County\tH1\n68527\t31109\tLincoln\tNE\tLancaster County\tH1\n68003\t31109\tAshland\tNE\tLancaster County\tH1\n68404\t31109\tMartell\tNE\tLancaster County\tH1\n68517\t31109\tLincoln\tNE\tLancaster County\tH1\n68529\t31109\tLincoln\tNE\tLancaster County\tH1\n68372\t31109\tHickman\tNE\tLancaster County\tH1\n68462\t31109\tWaverly\tNE\tLancaster County\tH1\n68333\t31109\tCrete\tNE\tLancaster County\tH1\n68402\t31109\tMalcolm\tNE\tLancaster County\tH1\n68524\t31109\tLincoln\tNE\tLancaster County\tH1\n68512\t31109\tLincoln\tNE\tLancaster County\tH1\n68465\t31109\tWilber\tNE\tLancaster County\tH1\n68317\t31109\tBennet\tNE\tLancaster County\tH1\n68358\t31109\tFirth\tNE\tLancaster County\tH1\n68514\t31109\tLincoln\tNE\tLancaster County\tH1\n68504\t31109\tLincoln\tNE\tLancaster County\tH1\n68505\t31109\tLincoln\tNE\tLancaster County\tH1\n68366\t31109\tGreenwood\tNE\tLancaster County\tH1\n68521\t31109\tLincoln\tNE\tLancaster County\tH1\n68532\t31109\tLincoln\tNE\tLancaster County\tH1\n68508\t31109\tLincoln\tNE\tLancaster County\tH1\n68520\t31109\tLincoln\tNE\tLancaster County\tH1\n68430\t31109\tRoca\tNE\tLancaster County\tH1\n68461\t31109\tWalton\tNE\tLancaster County\tH1\n68531\t31109\tLincoln\tNE\tLancaster County\tH1\n68336\t31109\tDavey\tNE\tLancaster County\tH1\n68542\t31109\tLincoln\tNE\tLancaster County\tH1\n69029\t31111\tFarnam\tNE\tLincoln County\tH1\n69101\t31111\tNorth platte\tNE\tLincoln County\tH1\n69138\t31111\tGothenburg\tNE\tLincoln County\tH1\n69038\t31111\tMaywood\tNE\tLincoln County\tH1\n69039\t31111\tMoorefield\tNE\tLincoln County\tH1\n69169\t31111\tWallace\tNE\tLincoln County\tH1\n69123\t31111\tBrady\tNE\tLincoln County\tH1\n69170\t31111\tWellfleet\tNE\tLincoln County\tH1\n69165\t31111\tSutherland\tNE\tLincoln County\tH1\n69103\t31111\tNorth platte\tNE\tLincoln County\tH1\n69120\t31111\tArnold\tNE\tLincoln County\tH1\n69143\t31111\tHershey\tNE\tLincoln County\tH1\n69163\t31111\tStapleton\tNE\tLincoln County\tH1\n69151\t31111\tMaxwell\tNE\tLincoln County\tH1\n69132\t31111\tDickens\tNE\tLincoln County\tH1\n69025\t31111\tCurtis\tNE\tLincoln County\tH1\n69120\t31113\tArnold\tNE\tLogan County\tH1\n69163\t31113\tStapleton\tNE\tLogan County\tH1\n68879\t31115\tTaylor\tNE\tLoup County\tH1\n68874\t31115\tSargent\tNE\tLoup County\tH1\n68813\t31115\tAnselmo\tNE\tLoup County\tH1\n68823\t31115\tBurwell\tNE\tLoup County\tH1\n69101\t31117\tNorth platte\tNE\tMcPherson County\tH1\n69155\t31117\tPaxton\tNE\tMcPherson County\tH1\n69165\t31117\tSutherland\tNE\tMcPherson County\tH1\n69163\t31117\tStapleton\tNE\tMcPherson County\tH1\n69167\t31117\tTryon\tNE\tMcPherson County\tH1\n68702\t31119\tNorfolk\tNE\tMadison County\tH1\n68781\t31119\tTilden\tNE\tMadison County\tH1\n68642\t31119\tHumphrey\tNE\tMadison County\tH1\n68748\t31119\tMadison\tNE\tMadison County\tH1\n68701\t31119\tNorfolk\tNE\tMadison County\tH1\n68644\t31119\tLindsay\tNE\tMadison County\tH1\n68752\t31119\tMeadow grove\tNE\tMadison County\tH1\n68715\t31119\tBattle creek\tNE\tMadison County\tH1\n68758\t31119\tNewman grove\tNE\tMadison County\tH1\n68826\t31121\tCentral city\tNE\tMerrick County\tH1\n68816\t31121\tArcher\tNE\tMerrick County\tH1\n68827\t31121\tChapman\tNE\tMerrick County\tH1\n68864\t31121\tPalmer\tNE\tMerrick County\tH1\n68628\t31121\tClarks\tNE\tMerrick County\tH1\n68663\t31121\tSilver creek\tNE\tMerrick County\tH1\n68638\t31121\tFullerton\tNE\tMerrick County\tH1\n68872\t31121\tSaint libory\tNE\tMerrick County\tH1\n68801\t31121\tGrand island\tNE\tMerrick County\tH1\n68640\t31121\tGenoa\tNE\tMerrick County\tH1\n69301\t31123\tAlliance\tNE\tMorrill County\tH1\n69148\t31123\tLisco\tNE\tMorrill County\tH1\n69125\t31123\tBroadwater\tNE\tMorrill County\tH1\n69336\t31123\tBridgeport\tNE\tMorrill County\tH1\n69331\t31123\tAngora\tNE\tMorrill County\tH1\n69334\t31123\tBayard\tNE\tMorrill County\tH1\n69131\t31123\tDalton\tNE\tMorrill County\tH1\n68864\t31125\tPalmer\tNE\tNance County\tH1\n68628\t31125\tClarks\tNE\tNance County\tH1\n68623\t31125\tBelgrade\tNE\tNance County\tH1\n68660\t31125\tSaint edward\tNE\tNance County\tH1\n68663\t31125\tSilver creek\tNE\tNance County\tH1\n68638\t31125\tFullerton\tNE\tNance County\tH1\n68627\t31125\tCedar rapids\tNE\tNance County\tH1\n68640\t31125\tGenoa\tNE\tNance County\tH1\n68882\t31125\tWolbach\tNE\tNance County\tH1\n68305\t31127\tAuburn\tNE\tNemaha County\tH1\n68378\t31127\tJohnson\tNE\tNemaha County\tH1\n68321\t31127\tBrownville\tNE\tNemaha County\tH1\n68379\t31127\tJulian\tNE\tNemaha County\tH1\n68421\t31127\tPeru\tNE\tNemaha County\tH1\n68376\t31127\tHumboldt\tNE\tNemaha County\tH1\n68442\t31127\tStella\tNE\tNemaha County\tH1\n68437\t31127\tShubert\tNE\tNemaha County\tH1\n68320\t31127\tBrock\tNE\tNemaha County\tH1\n68447\t31127\tTable rock\tNE\tNemaha County\tH1\n68348\t31127\tElk creek\tNE\tNemaha County\tH1\n68414\t31127\tNemaha\tNE\tNemaha County\tH1\n68448\t31127\tTalmage\tNE\tNemaha County\tH1\n68957\t31129\tLawrence\tNE\tNuckolls County\tH1\n68943\t31129\tHardy\tNE\tNuckolls County\tH1\n68325\t31129\tByron\tNE\tNuckolls County\tH1\n68935\t31129\tEdgar\tNE\tNuckolls County\tH1\n68974\t31129\tRuskin\tNE\tNuckolls County\tH1\n68964\t31129\tOak\tNE\tNuckolls County\tH1\n68942\t31129\tGuide rock\tNE\tNuckolls County\tH1\n68961\t31129\tNelson\tNE\tNuckolls County\tH1\n68934\t31129\tDeweese\tNE\tNuckolls County\tH1\n68978\t31129\tSuperior\tNE\tNuckolls County\tH1\n68938\t31129\tFairfield\tNE\tNuckolls County\tH1\n68335\t31129\tDavenport\tNE\tNuckolls County\tH1\n68410\t31131\tNebraska city\tNE\tOtoe County\tH1\n68301\t31131\tAdams\tNE\tOtoe County\tH1\n68329\t31131\tCook\tNE\tOtoe County\tH1\n68379\t31131\tJulian\tNE\tOtoe County\tH1\n68443\t31131\tSterling\tNE\tOtoe County\tH1\n68382\t31131\tLorton\tNE\tOtoe County\tH1\n68421\t31131\tPeru\tNE\tOtoe County\tH1\n68347\t31131\tEagle\tNE\tOtoe County\tH1\n68454\t31131\tUnadilla\tNE\tOtoe County\tH1\n68324\t31131\tBurr\tNE\tOtoe County\tH1\n68346\t31131\tDunbar\tNE\tOtoe County\tH1\n68320\t31131\tBrock\tNE\tOtoe County\tH1\n68446\t31131\tSyracuse\tNE\tOtoe County\tH1\n68317\t31131\tBennet\tNE\tOtoe County\tH1\n68413\t31131\tNehawka\tNE\tOtoe County\tH1\n68344\t31131\tDouglas\tNE\tOtoe County\tH1\n68417\t31131\tOtoe\tNE\tOtoe County\tH1\n68455\t31131\tUnion\tNE\tOtoe County\tH1\n68418\t31131\tPalmyra\tNE\tOtoe County\tH1\n68307\t31131\tAvoca\tNE\tOtoe County\tH1\n68448\t31131\tTalmage\tNE\tOtoe County\tH1\n68461\t31131\tWalton\tNE\tOtoe County\tH1\n68458\t31133\tVirginia\tNE\tPawnee County\tH1\n68323\t31133\tBurchard\tNE\tPawnee County\tH1\n68345\t31133\tDu bois\tNE\tPawnee County\tH1\n68441\t31133\tSteinauer\tNE\tPawnee County\tH1\n68376\t31133\tHumboldt\tNE\tPawnee County\tH1\n68381\t31133\tLiberty\tNE\tPawnee County\tH1\n68447\t31133\tTable rock\tNE\tPawnee County\tH1\n68420\t31133\tPawnee city\tNE\tPawnee County\tH1\n68348\t31133\tElk creek\tNE\tPawnee County\tH1\n68380\t31133\tLewiston\tNE\tPawnee County\tH1\n69169\t31135\tWallace\tNE\tPerkins County\tH1\n69155\t31135\tPaxton\tNE\tPerkins County\tH1\n69134\t31135\tElsie\tNE\tPerkins County\tH1\n69153\t31135\tOgallala\tNE\tPerkins County\tH1\n69033\t31135\tImperial\tNE\tPerkins County\tH1\n69122\t31135\tBig springs\tNE\tPerkins County\tH1\n69150\t31135\tMadrid\tNE\tPerkins County\tH1\n69140\t31135\tGrant\tNE\tPerkins County\tH1\n69168\t31135\tVenango\tNE\tPerkins County\tH1\n68845\t31137\tKearney\tNE\tPhelps County\tH1\n68924\t31137\tAxtell\tNE\tPhelps County\tH1\n68949\t31137\tHoldrege\tNE\tPhelps County\tH1\n68836\t31137\tElm creek\tNE\tPhelps County\tH1\n68940\t31137\tFunk\tNE\tPhelps County\tH1\n68863\t31137\tOverton\tNE\tPhelps County\tH1\n68923\t31137\tAtlanta\tNE\tPhelps County\tH1\n68982\t31137\tWilcox\tNE\tPhelps County\tH1\n68927\t31137\tBertrand\tNE\tPhelps County\tH1\n68958\t31137\tLoomis\tNE\tPhelps County\tH1\n68781\t31139\tTilden\tNE\tPierce County\tH1\n68769\t31139\tPlainview\tNE\tPierce County\tH1\n68786\t31139\tWausa\tNE\tPierce County\tH1\n68747\t31139\tMclean\tNE\tPierce County\tH1\n68738\t31139\tHadar\tNE\tPierce County\tH1\n68701\t31139\tNorfolk\tNE\tPierce County\tH1\n68765\t31139\tOsmond\tNE\tPierce County\tH1\n68752\t31139\tMeadow grove\tNE\tPierce County\tH1\n68771\t31139\tRandolph\tNE\tPierce County\tH1\n68767\t31139\tPierce\tNE\tPierce County\tH1\n68729\t31139\tCreighton\tNE\tPierce County\tH1\n68601\t31141\tColumbus\tNE\tPlatte County\tH1\n68653\t31141\tPlatte center\tNE\tPlatte County\tH1\n68642\t31141\tHumphrey\tNE\tPlatte County\tH1\n68748\t31141\tMadison\tNE\tPlatte County\tH1\n68647\t31141\tMonroe\tNE\tPlatte County\tH1\n68660\t31141\tSaint edward\tNE\tPlatte County\tH1\n68644\t31141\tLindsay\tNE\tPlatte County\tH1\n68602\t31141\tColumbus\tNE\tPlatte County\tH1\n68643\t31141\tLeigh\tNE\tPlatte County\tH1\n68631\t31141\tCreston\tNE\tPlatte County\tH1\n68634\t31141\tDuncan\tNE\tPlatte County\tH1\n68758\t31141\tNewman grove\tNE\tPlatte County\tH1\n68640\t31141\tGenoa\tNE\tPlatte County\tH1\n68601\t31143\tColumbus\tNE\tPolk County\tH1\n68654\t31143\tPolk\tNE\tPolk County\tH1\n68367\t31143\tGresham\tNE\tPolk County\tH1\n68628\t31143\tClarks\tNE\tPolk County\tH1\n68651\t31143\tOsceola\tNE\tPolk County\tH1\n68663\t31143\tSilver creek\tNE\tPolk County\tH1\n68316\t31143\tBenedict\tNE\tPolk County\tH1\n68658\t31143\tRising city\tNE\tPolk County\tH1\n68666\t31143\tStromsburg\tNE\tPolk County\tH1\n68662\t31143\tShelby\tNE\tPolk County\tH1\n69024\t31145\tCulbertson\tNE\tRed Willow County\tH1\n69026\t31145\tDanbury\tNE\tRed Willow County\tH1\n69001\t31145\tMc cook\tNE\tRed Willow County\tH1\n69022\t31145\tCambridge\tNE\tRed Willow County\tH1\n69046\t31145\tWilsonville\tNE\tRed Willow County\tH1\n69020\t31145\tBartley\tNE\tRed Willow County\tH1\n69034\t31145\tIndianola\tNE\tRed Willow County\tH1\n69036\t31145\tLebanon\tNE\tRed Willow County\tH1\n68431\t31147\tRulo\tNE\tRichardson County\tH1\n68345\t31147\tDu bois\tNE\tRichardson County\tH1\n68376\t31147\tHumboldt\tNE\tRichardson County\tH1\n68442\t31147\tStella\tNE\tRichardson County\tH1\n68437\t31147\tShubert\tNE\tRichardson County\tH1\n68355\t31147\tFalls city\tNE\tRichardson County\tH1\n68457\t31147\tVerdon\tNE\tRichardson County\tH1\n68433\t31147\tSalem\tNE\tRichardson County\tH1\n68337\t31147\tDawson\tNE\tRichardson County\tH1\n68759\t31149\tNewport\tNE\tRock County\tH1\n68823\t31149\tBurwell\tNE\tRock County\tH1\n68714\t31149\tBassett\tNE\tRock County\tH1\n69217\t31149\tLong pine\tNE\tRock County\tH1\n68464\t31151\tWestern\tNE\tSaline County\tH1\n68339\t31151\tDenton\tNE\tSaline County\tH1\n68406\t31151\tMilligan\tNE\tSaline County\tH1\n68423\t31151\tPleasant dale\tNE\tSaline County\tH1\n68343\t31151\tDorchester\tNE\tSaline County\tH1\n68359\t31151\tFriend\tNE\tSaline County\tH1\n68341\t31151\tDe witt\tNE\tSaline County\tH1\n68333\t31151\tCrete\tNE\tSaline County\tH1\n68405\t31151\tMilford\tNE\tSaline County\tH1\n68465\t31151\tWilber\tNE\tSaline County\tH1\n68453\t31151\tTobias\tNE\tSaline County\tH1\n68445\t31151\tSwanton\tNE\tSaline County\tH1\n68424\t31151\tPlymouth\tNE\tSaline County\tH1\n68338\t31151\tDaykin\tNE\tSaline County\tH1\n68059\t31153\tSpringfield\tNE\tSarpy County\tH1\n68138\t31153\tOmaha\tNE\tSarpy County\tH1\n68197\t31153\tOmaha\tNE\tSarpy County\tH1\n68136\t31153\tOmaha\tNE\tSarpy County\tH1\n68069\t31153\tWaterloo\tNE\tSarpy County\tH1\n68133\t31153\tPapillion\tNE\tSarpy County\tH1\n68046\t31153\tPapillion\tNE\tSarpy County\tH1\n68147\t31153\tBellevue\tNE\tSarpy County\tH1\n68113\t31153\tOffutt afb\tNE\tSarpy County\tH1\n68056\t31153\tSt columbans\tNE\tSarpy County\tH1\n68123\t31153\tBellevue\tNE\tSarpy County\tH1\n68028\t31153\tGretna\tNE\tSarpy County\tH1\n68128\t31153\tLa vista\tNE\tSarpy County\tH1\n68157\t31153\tOmaha\tNE\tSarpy County\tH1\n68005\t31153\tBellevue\tNE\tSarpy County\tH1\n68050\t31155\tPrague\tNE\tSaunders County\tH1\n68036\t31155\tLinwood\tNE\tSaunders County\tH1\n68626\t31155\tBrainard\tNE\tSaunders County\tH1\n68070\t31155\tWeston\tNE\tSaunders County\tH1\n68017\t31155\tCeresco\tNE\tSaunders County\tH1\n68648\t31155\tMorse bluff\tNE\tSaunders County\tH1\n68018\t31155\tColon\tNE\tSaunders County\tH1\n68041\t31155\tMead\tNE\tSaunders County\tH1\n68015\t31155\tCedar bluffs\tNE\tSaunders County\tH1\n68042\t31155\tMemphis\tNE\tSaunders County\tH1\n68033\t31155\tIthaca\tNE\tSaunders County\tH1\n68064\t31155\tValley\tNE\tSaunders County\tH1\n68073\t31155\tYutan\tNE\tSaunders County\tH1\n68065\t31155\tValparaiso\tNE\tSaunders County\tH1\n68025\t31155\tFremont\tNE\tSaunders County\tH1\n68003\t31155\tAshland\tNE\tSaunders County\tH1\n68066\t31155\tWahoo\tNE\tSaunders County\tH1\n68040\t31155\tMalmo\tNE\tSaunders County\tH1\n68001\t31155\tAbie\tNE\tSaunders County\tH1\n68366\t31155\tGreenwood\tNE\tSaunders County\tH1\n69358\t31157\tMorrill\tNE\tScotts Bluff County\tH1\n69357\t31157\tMitchell\tNE\tScotts Bluff County\tH1\n69361\t31157\tScottsbluff\tNE\tScotts Bluff County\tH1\n69352\t31157\tLyman\tNE\tScotts Bluff County\tH1\n69356\t31157\tMinatare\tNE\tScotts Bluff County\tH1\n69353\t31157\tMcgrew\tNE\tScotts Bluff County\tH1\n69355\t31157\tMelbeta\tNE\tScotts Bluff 
